vi "Histogram of timing data.vi"() -> ()   [LabVIEW 2013]
uses:
  GP22_TDC_Arduinoed.lvlib
panel:
  out "Timing histogram":cluster{"Bins":dbl[], "Binned data":i32[]}(graph)
  out "error out":errorcluster
  in  "VISA resource name":refnum<visa-resource-name>
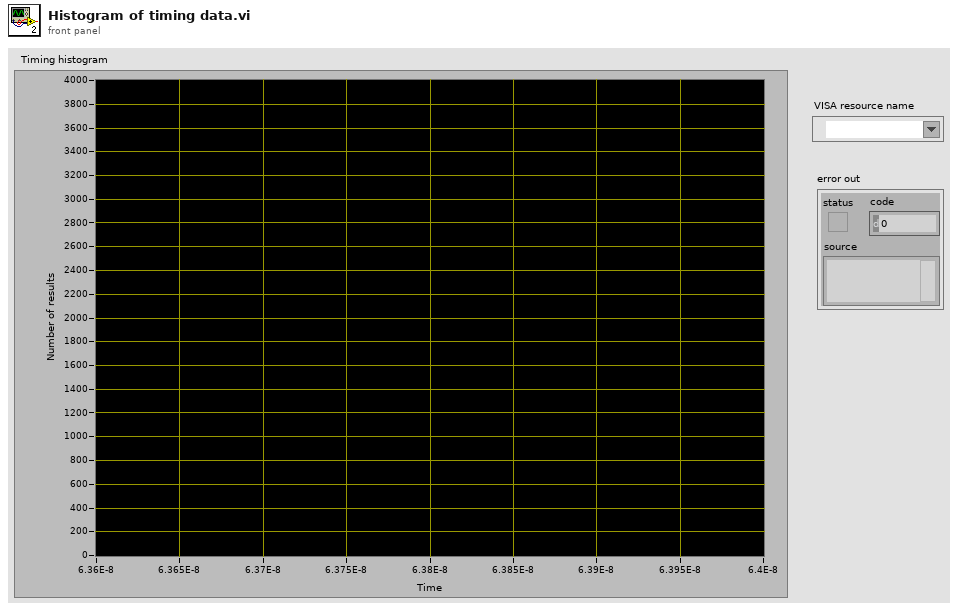
[diagram p1: front panel]
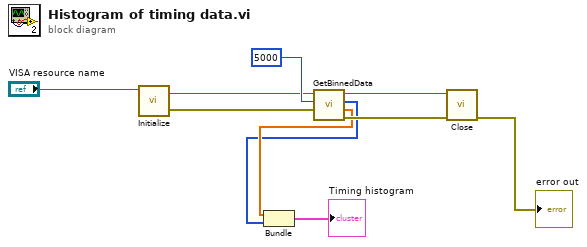
[diagram p0: block diagram]
diagram:
  n1 = call "Initialize.vi"("VISA resource name"="VISA resource name") -> ("error out"=w6:errorcluster, "VISA resource name out"=w8:refnum<visa-resource-name>)  [unwired: 5 in]
  n2 = call "GetBinnedData.vi"("error in"=w6, "Time in ms (30000)"=u32 5000, "VISA resource name"=w8) -> ("error out"=w5:errorcluster, "Bins"=w3:dbl[], "Binned data"=w2:i32[], "VISA resource name out"=w7:refnum<visa-resource-name>)  [unwired: 5 in]
  n3 = Bundle("Bins"=w3, "Binned data"=w2) -> (→"Timing histogram":cluster{"Bins":dbl[], "Binned data":i32[]})  [unwired: 1 in]
  n4 = call "Close.vi"("error in (no error)"=w5, "VISA resource name"=w7) -> ("error out"=→"error out":errorcluster)  [unwired: 9 in]
